vi "Create_Raw_data_file.vi"(4 "No of averages":i32=1, 5 "End time":dbl, 6 "Start time":dbl, 7 "Setup filename":string) -> (0 "Error String":string, 1 "Values":string[][](array[string]), 2 "Header Comments":string[](array[string]), 3 "Column headers":string[](array[string]))   [LabVIEW 2011]
uses:
  File/Setup_Filetype.ctl
  Controls/Post_Process.ctl
  Globals/Preference_global.vi
  Globals/Meas_global.vi
  Globals/Trav_pos_global.vi
  Globals/Constants_global.vi
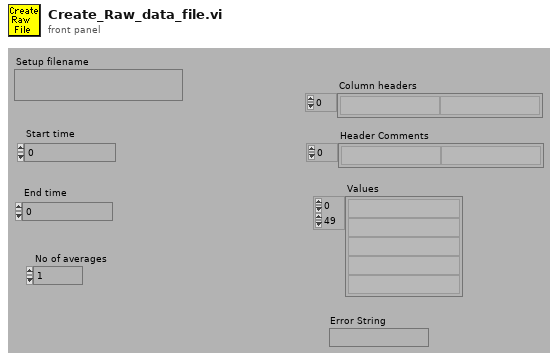
[diagram p1: front panel]
types:
  T1 = typedef "Post_Process.ctl" = enum16{"Take New Data", "Post Process Raw Data File"}
  T2 = typedef "Server_Comms.ctl" = enum16{"Server Link Healthy", "Do Not Link To Server"}
  T3 = typedef "Setup_Filetype.ctl" = enum16{"Measurement Setups", "Calibration Setups", "General", "Results File Plotter Setups", "Speed Calib Tweaks"}
  T4 = typedef "Traverse_cluster.ctl" = cluster{"Start X":dbl, "Start Y":dbl, "Start Z":dbl, "End X":dbl, "End Y":dbl, "End Z":dbl, "No. of pts.":i32, "Spacing":T5, "Filename":path, "Tunnel Speed":dbl, "Averaging time (min)":dbl, "Extra Commands":string, "Specific Arguments":string, "Emission Rate (l/min)":dbl, "Trace Gas Concentration (%)":dbl, "Density Ratio":string, "Comments":string, "Row No":i32, "Row Type Selector":T6, "Completion time":string, "Row Duration (mins)":dbl, "No. of Valid pts.":i32, "Meas Setup File":string}
  T5 = typedef "Spacing.ctl" = enum16{"Linear", "Log", "Gauss", "Specified", "N/A"}
  T6 = typedef "Multi_run_mode.ctl" = enum16{"Move Traverse Only", "Set Tunnel Speed Only", "Set Source Only", "Set Measurement Conditions", "Single Measurement", "Vertical Profile", "Lateral Profile", "Longitudinal Profile", "Explore Volume", "Multi-Axis Profile", "Auto Calibrate", "Meas Fast FID Bkgnd", "Check Beam Power", "Scanning Valve Measurement", "Run VI Named:", "Set ADAM Ch", "Wait (minutes)", "Send Message", "Synchronize With:", "Fall Back to this Row", "Turn Off Row Repeating", "Blank Row"}
  T7 = cluster{"Name":string, "X":dbl, "Y":dbl, "Z":dbl}[]
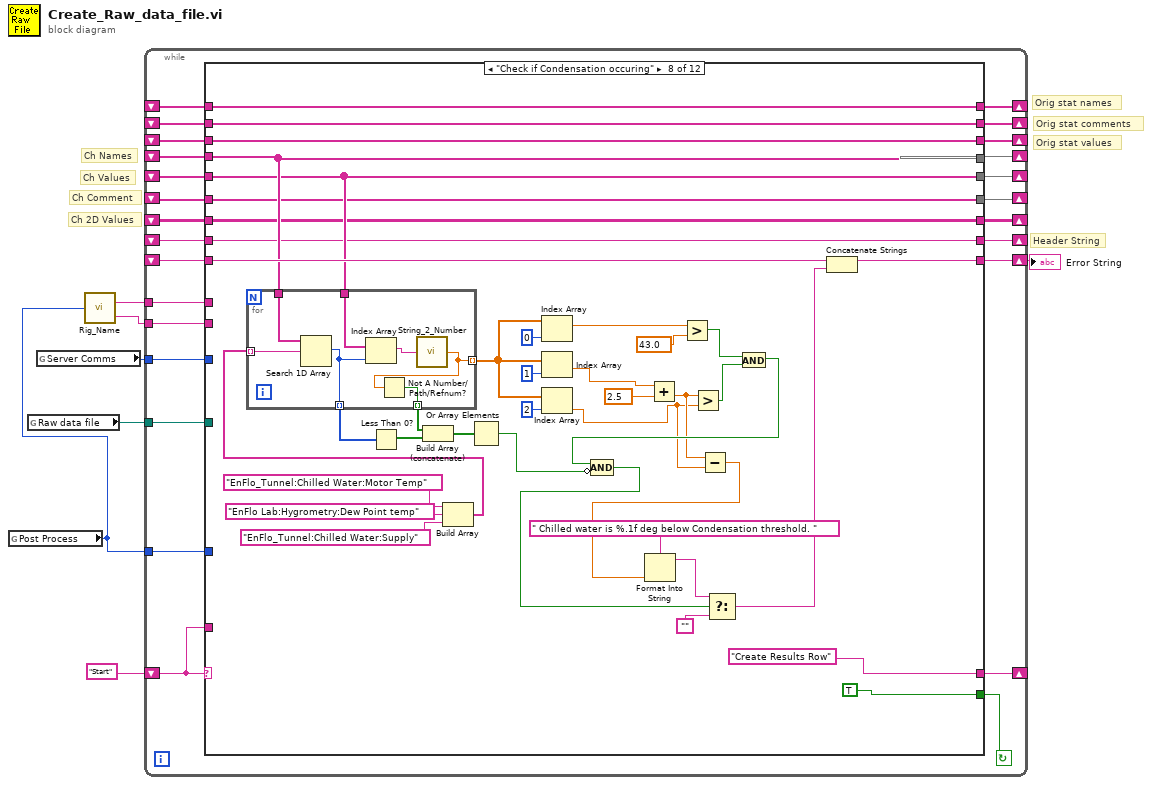
[diagram p0: block diagram]
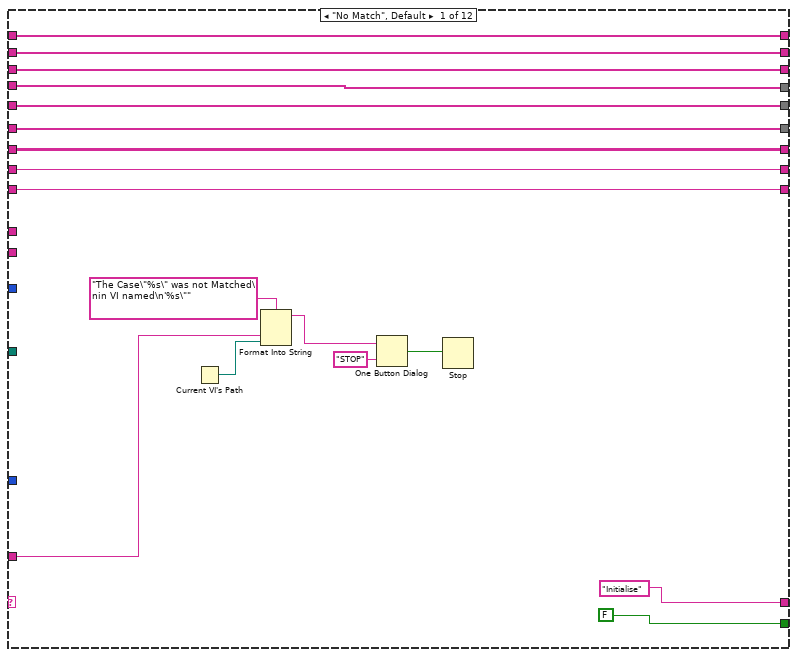
[diagram p2: hidden frame]
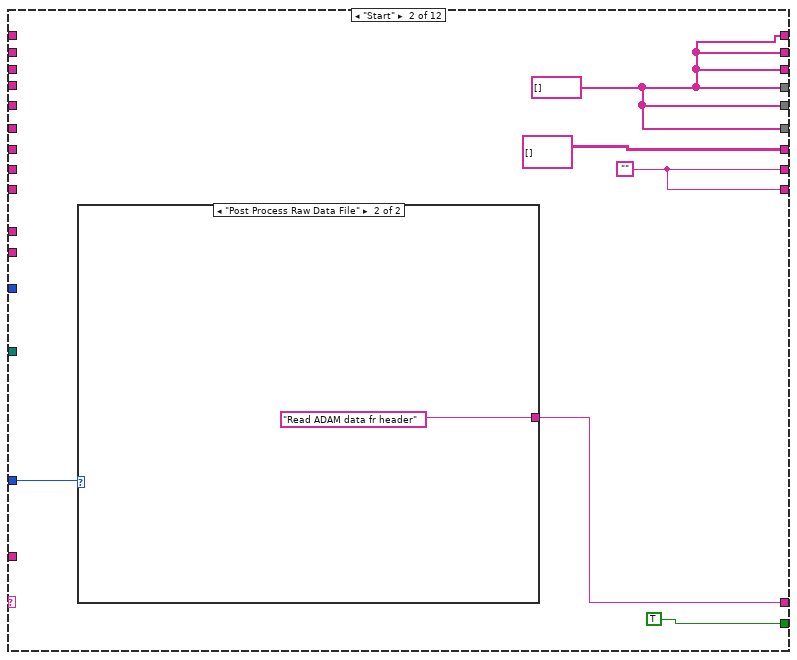
[diagram p3: hidden frame]
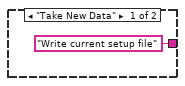
[diagram p4: hidden frame]
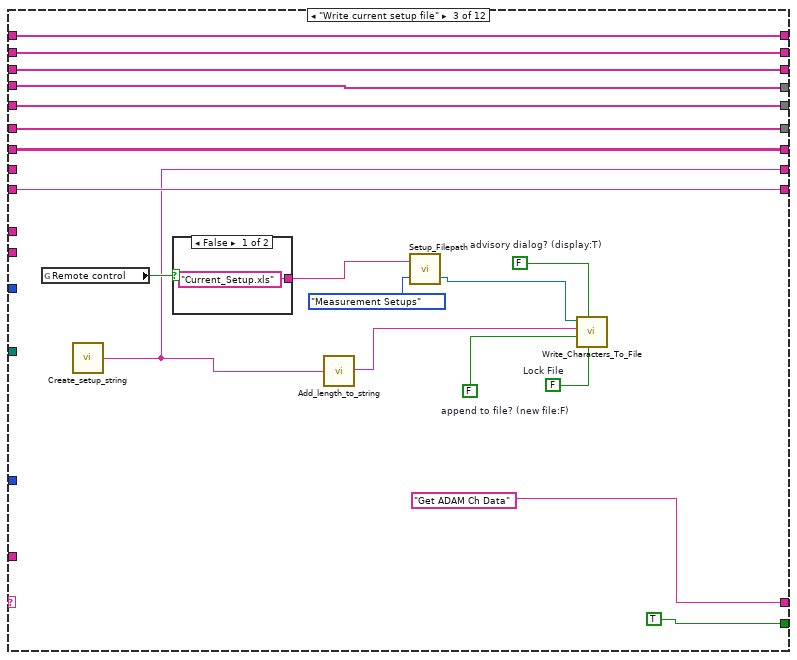
[diagram p5: hidden frame]
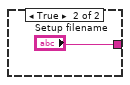
[diagram p6: hidden frame]
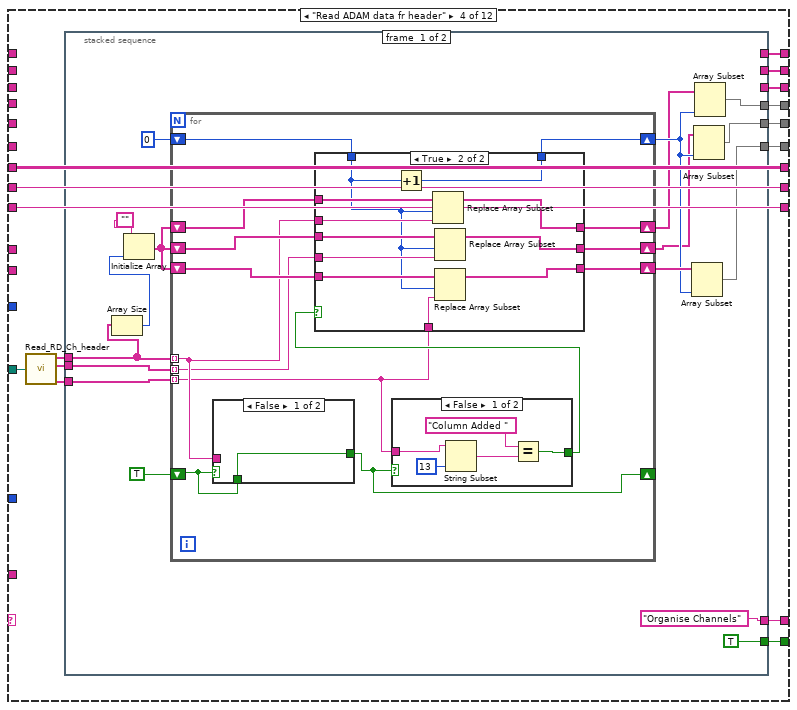
[diagram p7: hidden frame]
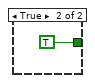
[diagram p9: hidden frame]
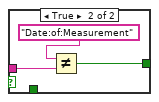
[diagram p10: hidden frame]
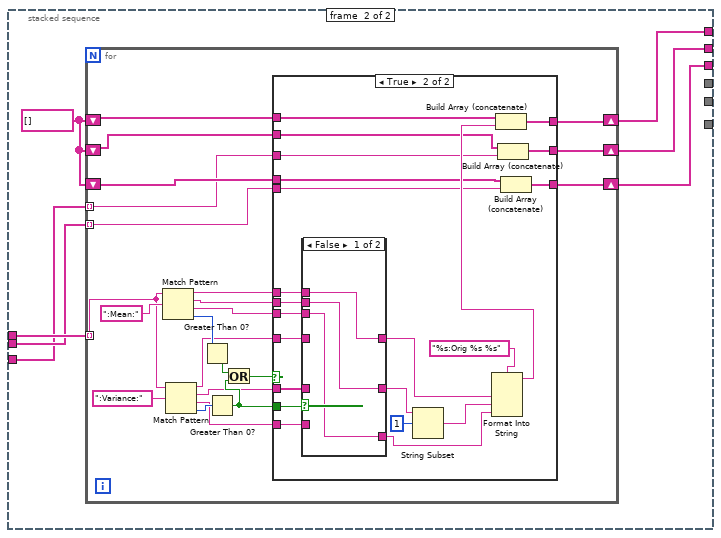
[diagram p11: hidden frame]
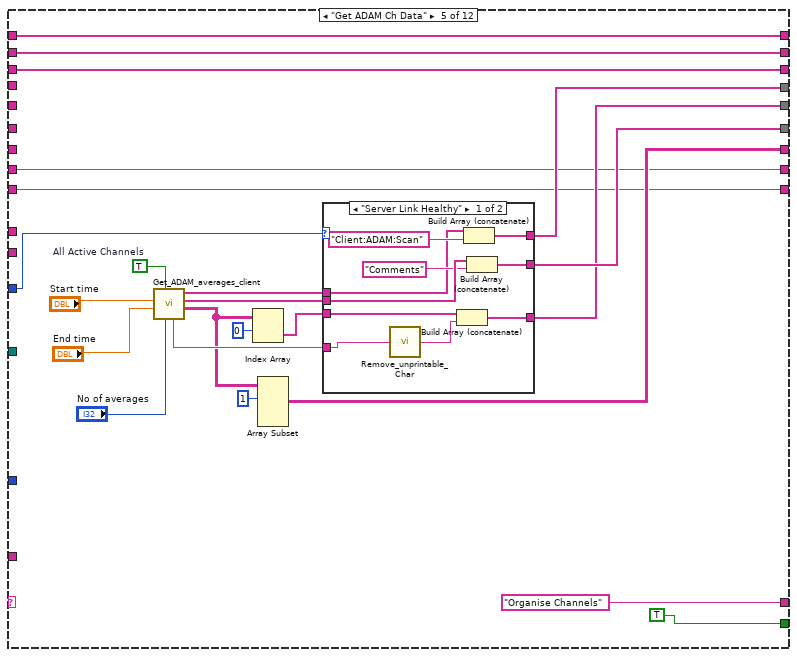
[diagram p14: hidden frame]
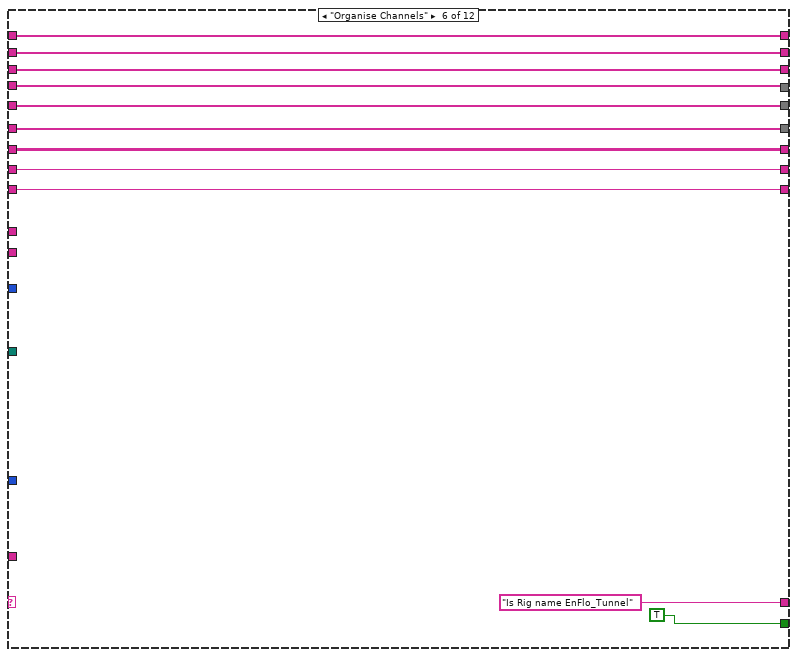
[diagram p16: hidden frame]
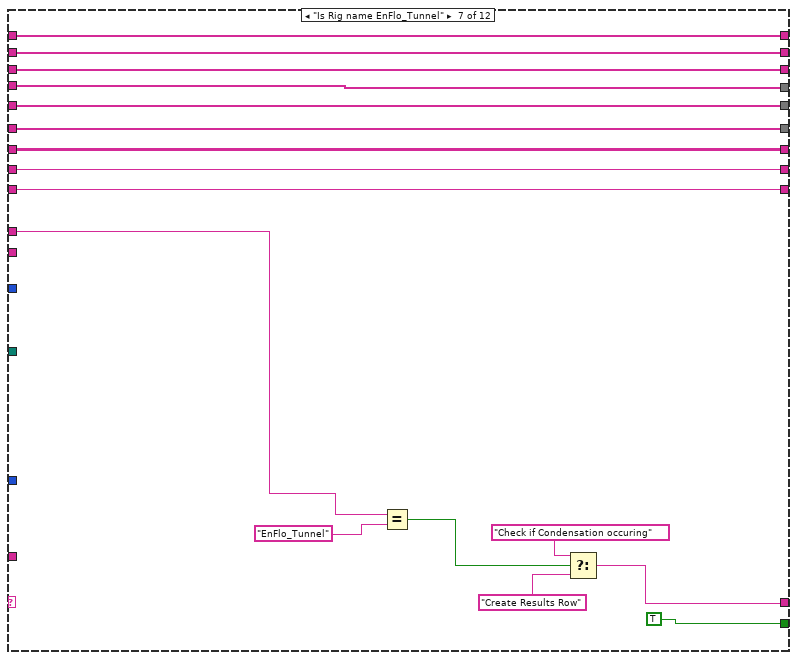
[diagram p17: hidden frame]
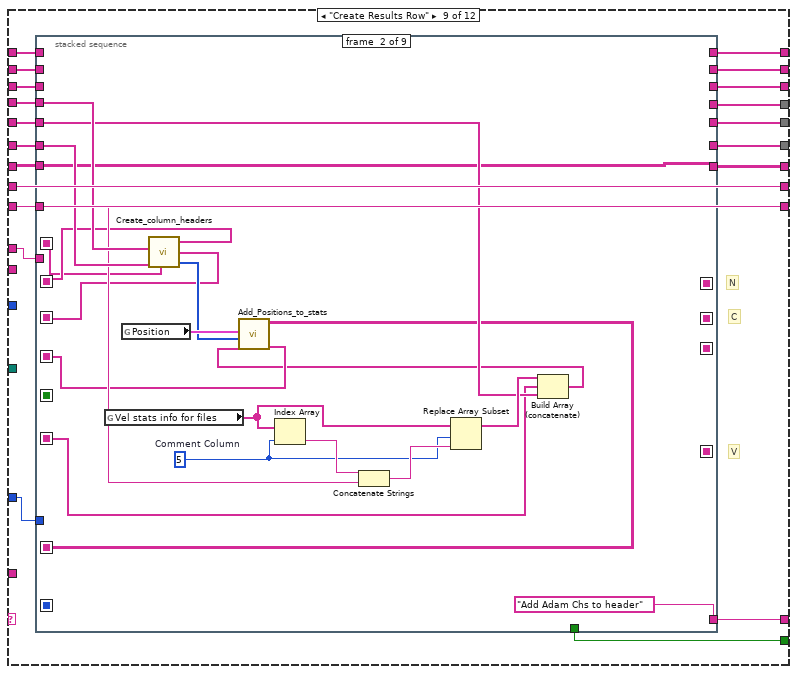
[diagram p18: hidden frame]
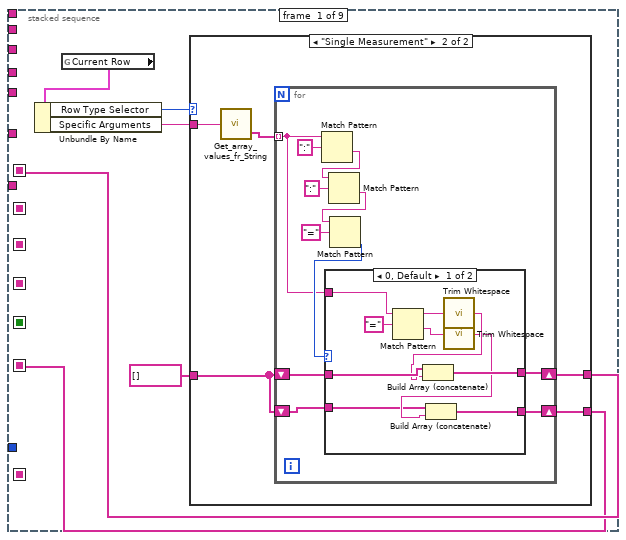
[diagram p19: hidden frame]
diagram:
  # "Orig stat values"
  # "Orig stat comments"
  # "Orig stat names"
  # "Header String"
  # "Ch 2D Values"
  # "Ch Comment"
  # "Ch Values"
  # "Ch Names"
  n1 = global read "Meas_global.vi" "Post Process"() -> (w3:T1)
  n2 = global read "Meas_global.vi" "Raw data file"() -> (w6:path)
  n3 = global read "Preference_global.vi" "Server Comms"() -> (w5:T2)
  n4 = call "Rig_Name.vi"("Post Process"=w3) -> ("Rig Setup before dash"=w2:string, "Hard Disk name"=w1:string)
  n5 = while {
    tunnel: w5 -> [w16]
    tunnel: w6 -> [w17]
    tunnel: w3 -> [w18]
    shift-left: _ -> [w20]
    shift-right: [w19] -> _
    shift-left: _ -> [w26]
    shift-right: [w25] -> w4
    shift-left: _ -> [w21]
    shift-right: [w27] -> _
    shift-left: _ -> [w22]
    shift-right: [w29] -> _
    shift-left: _ -> [w23]
    shift-right: [w28] -> _
    shift-left: _ -> [w24]
    shift-right: [w30] -> _
    shift-left: "Start" -> [w31]
    shift-right: [w32] -> _
    tunnel: w2 -> [w15]
    tunnel: w1 -> [w14]
    shift-right: [w10] -> _
    shift-left: _ -> [w11]
    shift-right: [w8] -> _
    shift-left: _ -> [w9]
    shift-right: [w12] -> _
    shift-left: _ -> [w13]
    stop <- w33 continue-if-true
    n6 = case shown="\"Check if Condensation occuring\"" w31 {
      tunnel: [FALSE TRUE TRUE w83 TRUE TRUE TRUE TRUE w328 TRUE TRUE FALSE] -> w33
      tunnel: ["Initialise" w52 "Get ADAM Ch Data" w94 "Organise Channels" "Is Rig name EnFlo_Tunnel" w265 "Create Results Row" w340 "Add Raw Data header info" "Add Raw Data fr Tempory file" "End"] -> w32
      tunnel: w31 -> [w45 _ _ _ _ _ _ _ _ _ _ _]
      tunnel: [w42 w51 w77 w85 w221 w255 w273 w283 w337 w610 w640 w657] -> w30
      tunnel: [w40 w51 w75 w86 w220 w253 w271 w281 w334 w621 w642 w659] -> w29
      tunnel: [w41 w51 w76 w84 w219 w254 w272 w282 w330 w622 w641 w658] -> w28
      tunnel: [w39 string[][] [] w74 w92 w217 w252 w270 w280 w332 w613 w643 w660] -> w27
      tunnel: w26 -> [w38 _ w72 w93 w216 w250 w267 w286 w338 w626 w644 w661]
      tunnel: [w38 w54 w72 w93 w216 w250 w267 w284 w338 w626 w644 w661] -> w25
      tunnel: w24 -> [w42 _ w77 _ _ w255 w273 w283 w336 w610 w640 w657]
      tunnel: w23 -> [w41 _ w76 _ _ w254 w272 w282 w331 w622 w641 w658]
      tunnel: w22 -> [w40 _ w75 _ _ w253 w271 w281 w335 w621 w642 w659]
      tunnel: w21 -> [w39 _ w74 w92 _ w252 w270 w280 w333 w613 w643 w660]
      tunnel: w20 -> [w37 _ _ w91 w215 w251 w268 w278 w339 w615 w637 w656]
      tunnel: [w37 w54 w66 w91 w215 w251 w268 w278 w339 w618 w636 ""] -> w19
      tunnel: w18 -> [_ w53 _ _ _ _ _ _ w329 _ _ _]
      tunnel: w17 -> [_ _ _ w90 _ _ _ _ _ _ _ w652]
      tunnel: w16 -> [_ _ _ _ w214 _ _ _ _ _ _ _]
      tunnel: w15 -> [_ _ _ _ _ _ w262 _ w327 _ _ _]
      tunnel: w14 -> [_ _ _ _ _ _ _ _ _ _ _ _]
      tunnel: w13 -> [w36 _ w64 _ w213 w249 w260 w277 w325 w607 w635 w649]
      tunnel: [w36 w51 w64 w82 w213 w249 w260 w277 w326 w607 w635 w649] -> w12
      tunnel: w11 -> [w35 _ w63 _ w212 w248 w259 w276 w324 w606 w634 w648]
      tunnel: [w35 w51 w63 w81 w212 w248 w259 w276 w323 w606 w634 w648] -> w10
      tunnel: w9 -> [w34 _ w62 _ w211 w247 w258 w275 w321 w605 w633 w647]
      tunnel: [w34 w51 w62 w80 w211 w247 w258 w275 w322 w605 w633 w647] -> w8
      frame "No Match", Default {
        n7 = Current VI's Path() -> (path=w44:path)
        n8 = Format Into String(format string="The Case\"%s\" was not Matched\nin VI named\n'%s\"" ("Format String"), w45, w44) -> (resulting string=w48:string)  [unwired: 2 in, 1 out]
        n9 = One Button Dialog(message=w48, button name ("OK")="STOP") -> (true=w46:bool)
        n10 = Stop(stop? (T)=w46) -> ()
      }
      frame "Start" {
        w54 = ""
        w51 = string[] []
        n11 = case shown="\"Post Process Raw Data File\"" w53 {
          tunnel: ["Write current setup file" "Read ADAM data fr header"] -> w52
          frame "Take New Data" {
          }
          frame "Post Process Raw Data File" {
          }
        }
      }
      frame "Write current setup file" {
        w67 = FALSE  # Lock File
        w70 = FALSE  # advisory dialog? (display:T)
        w71 = FALSE  # append to file? (new file:F)
        n12 = global read "Meas_global.vi" "Remote control"() -> (w69:bool)
        n13 = call "Create_setup_string.vi"() -> ("Setup String"=w66:string)  [unwired: 1 out]
        n14 = case shown="False" w69 {
          tunnel: ["Current_Setup.xls" ("Setup filename") "Setup filename"] -> w60
          frame False {
          }
          frame True {
          }
        }
        n15 = call "Add_length_to_string.vi"("String in"=w66) -> ("String out"=w68:string)
        n16 = call "Setup_Filepath.vi"("Setup File Type"=Setup_Filetype."Measurement Setups", "Filename in"=w60) -> ("Filename Out"=w59:path)  [unwired: 1 out]
        n17 = call "Write_Characters_To_File.vi"("file path (dialog if empty)"=w59, "advisory dialog? (display:T)"=w70, "character string"=w68, "append to file? (new file:F)"=w71, "Lock File"=w67) -> ()  [unwired: 4 out]
      }
      frame "Read ADAM data fr header" {
        n18 = call "Read_RD_Ch_header.vi"("Raw data file"=w90) -> ("Ch Name Out"=w88:string[], "Ch Values"=w87:string[], "Comments"=w89:string[])  [unwired: 1 out]
        n19 = stacked-sequence {
          tunnel: ["Organise Channels" _] -> w94
          tunnel: w89 -> [w109 w154]
          tunnel: w88 -> [w108 w157]
          tunnel: w87 -> [w103 w155]
          tunnel: [w100 _] -> w86
          tunnel: [w97 _] -> w85
          tunnel: [w96 _] -> w84
          tunnel: [TRUE _] -> w83
          tunnel: [_ w153] -> w82
          tunnel: [_ w152] -> w81
          tunnel: [_ w151] -> w80
          frame #0 {
            n20 = Array Size(array=w108) -> (size(s)=w106:i32)
            n21 = Initialize Array("", w106) -> (w105:string[])
            n22 = for {
              shift-right: [w112] -> w101
              shift-left: 0 -> [w122]
              shift-right: [w116] -> w102
              shift-left: w105 -> [w119]
              shift-right: [w117] -> w99
              shift-left: w105 -> [w120]
              shift-right: [w118] -> w98
              shift-left: w105 -> [w121]
              shift-right: [w124] -> _
              shift-left: TRUE -> [w125]
              tunnel: w108 -> [w115] mode=indexing
              tunnel: w109 -> [w113] mode=indexing
              tunnel: w103 -> [w114] mode=indexing
              n23 = case shown="False" w125 {
                tunnel: w115 -> [_ w150]
                tunnel: [w147 w148] -> w124
                tunnel: w125 -> [w147 _]
                frame False {
                }
                frame True {
                  n24 = Not Equal?(x="Date:of:Measurement", y=w150) -> (x != y?=w148:bool)
                }
              }
              n25 = case shown="False" w124 {
                tunnel: w113 -> [w142 _]
                tunnel: [w144 TRUE] -> w123
                frame False {
                  n26 = String Subset(string=w142, length (rest)=13 ("length (rest)")) -> (substring=w141:string)  [unwired: 1 out]
                  n27 = Equal?(x="Column Added ", y=w141) -> (x = y?=w144:bool)
                }
                frame True {
                }
              }
              n28 = case shown="True" w123 {
                tunnel: w122 -> [w126 w131]
                tunnel: w121 -> [w129 w140]
                tunnel: w120 -> [w128 w139]
                tunnel: w119 -> [w127 w138]
                tunnel: [w129 w137] -> w118
                tunnel: [w128 w136] -> w117
                tunnel: [w127 w135] -> w116
                tunnel: w115 -> [_ w134]
                tunnel: w114 -> [_ w133]
                tunnel: w113 -> [_ w132]
                tunnel: [w126 w130] -> w112
                frame False {
                }
                frame True {
                  n29 = Increment(x=w131) -> (x+1=w130:i32)
                  n30 = Replace Array Subset(array=w140, new element=w134, index=w131) -> (w137:string[])
                  n31 = Replace Array Subset(array=w139, new element=w133, index=w131) -> (w136:string[])
                  n32 = Replace Array Subset(array=w138, new element=w132, index=w131) -> (w135:string[])
                }
              }
            }
            n33 = Array Subset(array=w102, length=w101) -> (w100:string[])  [unwired: 1 in]
            n34 = Array Subset(array=w99, length=w101) -> (w96:string[])  [unwired: 1 in]
            n35 = Array Subset(array=w98, length=w101) -> (w97:string[])  [unwired: 1 in]
          }
          frame #1 {
            w156 = string[] []
            n36 = for {
              shift-right: [w165] -> w153
              shift-left: w156 -> [w164]
              shift-right: [w158] -> w152
              shift-left: w156 -> [w159]
              shift-right: [w161] -> w151
              shift-left: w156 -> [w162]
              tunnel: w157 -> [w177] mode=indexing
              tunnel: w155 -> [w163] mode=indexing
              tunnel: w154 -> [w160] mode=indexing
              n37 = Match Pattern(string=w177, regular expression=":Mean:") -> (before substring=w168:string, match substring=w167:string, after substring=w166:string, offset past match=w176:i32)  [unwired: 1 out]
              n38 = Match Pattern(string=w177, regular expression=":Variance:") -> (before substring=w171:string, match substring=w170:string, after substring=w169:string, offset past match=w175:i32)  [unwired: 1 out]
              n39 = Greater Than 0?(x=w176) -> (x > 0?=w174:bool)
              n40 = Greater Than 0?(x=w175) -> (x > 0?=w172:bool)
              n41 = Or(x=w174, y=w172) -> (x .or. y?=w173:bool)
              n42 = case shown="True" w173 {
                tunnel: w172 -> [_ w204]
                tunnel: w171 -> [_ w203]
                tunnel: w170 -> [_ w202]
                tunnel: w169 -> [_ w201]
                tunnel: w168 -> [_ w194]
                tunnel: w167 -> [_ w193]
                tunnel: w166 -> [_ w192]
                tunnel: [w182 w190] -> w165
                tunnel: w164 -> [w182 w189]
                tunnel: w163 -> [_ w188]
                tunnel: w162 -> [w180 w187]
                tunnel: [w180 w186] -> w161
                tunnel: w160 -> [_ w185]
                tunnel: w159 -> [w181 w184]
                tunnel: [w181 w183] -> w158
                frame False {
                }
                frame True {
                  n43 = case shown="False" w204 {
                    tunnel: w203 -> [_ w209]
                    tunnel: w202 -> [_ w210]
                    tunnel: w201 -> [_ w208]
                    tunnel: [w206 w210] -> w199
                    tunnel: [w207 w209] -> w196
                    tunnel: [w205 w208] -> w195
                    tunnel: w194 -> [w207 _]
                    tunnel: w193 -> [w206 _]
                    tunnel: w192 -> [w205 _]
                    frame False {
                    }
                    frame True {
                    }
                  }
                  n44 = String Subset(string=w199, offset (0)=1) -> (substring=w198:string)  [unwired: 1 out]
                  n45 = Format Into String(format string="%s:Orig %s %s", w196, w198, w195) -> (resulting string=w191:string)  [unwired: 2 in, 1 out]
                  n46 = Build Array (concatenate)(w189, w191) -> (w190:string[])
                  n47 = Build Array (concatenate)(w184, w185) -> (w183:string[])
                  n48 = Build Array (concatenate)(w187, w188) -> (w186:string[])
                }
              }
            }
          }
        }
      }
      frame "Get ADAM Ch Data" {
        w224 = TRUE  # All Active Channels
        n49 = call "Get_ADAM_averages_client.vi"("No of averages"="No of averages", "All Active Channels"=w224, "End time"="End time", "Start time"="Start time") -> ("Values"=w227:string[][], "Comments"=w230:string[], "Titles"=w229:string[], "Messages"=w231:string)  [unwired: 1 in, 3 out]
        n50 = Index Array(array=w227, index (row)=0 ("Index")) -> (element=w218:string[])  [unwired: 1 in]
        n51 = Array Subset(array=w227, index (row)=1 ("Array Index")) -> (w217:string[][])  [unwired: 3 in]
        n52 = case shown="\"Server Link Healthy\"" w214 {
          tunnel: w231 -> [w235 _]
          tunnel: w230 -> [w243 w245]
          tunnel: w229 -> [w240 w246]
          tunnel: [w239 w246] -> w221
          tunnel: [w238 w245] -> w220
          tunnel: [w237 w244] -> w219
          tunnel: w218 -> [w236 w244]
          frame "Server Link Healthy" {
            n53 = call "Remove_unprintable_Char.vi"("Input String"=w235) -> ("Output String"=w234:string)
            n54 = Build Array (concatenate)(w236, w234) -> (w237:string[])
            n55 = Build Array (concatenate)(w240, "Client:ADAM:Scan") -> (w239:string[])
            n56 = Build Array (concatenate)(w243, "Comments" ("Comments")) -> (w238:string[])
          }
          frame "Do Not Link To Server" {
          }
        }
      }
      frame "Organise Channels" {
      }
      frame "Is Rig name EnFlo_Tunnel" {
        n57 = Equal?(x=w262, y="EnFlo_Tunnel") -> (x = y?=w266:bool)
        n58 = Select(t="Check if Condensation occuring", s=w266, f="Create Results Row") -> (s? t:f=w265:string)
      }
      frame "Check if Condensation occuring" {
        n59 = Build Array("EnFlo_Tunnel:Chilled Water:Motor Temp", "EnFlo Lab:Hygrometry:Dew Point temp", "EnFlo_Tunnel:Chilled Water:Supply") -> (w309:string[])
        n60 = for {
          tunnel: w283 -> [w320]
          tunnel: w309 -> [w319] mode=indexing
          tunnel: w282 -> [w318]
          tunnel: [w316] -> w310 mode=indexing
          tunnel: [w315] -> w308 mode=indexing
          tunnel: [w314] -> w301 mode=indexing
          n61 = Search 1D Array(1D array=w320, element=w319) -> (index of element=w316:i32)  [unwired: 1 out]
          n62 = Index Array(array=w318, index=w316) -> (element=w317:string)
          n63 = call "String_2_Number.vi"("Value"=w317) -> ("Numeric"=w315:dbl)
          n64 = Not A Number/Path/Refnum?(number/path/refnum=w315) -> (NaN/Path/Refnum?=w314:bool)
        }
        n65 = Less Than 0?(x=w310) -> (x < 0?=w300:bool[])
        n66 = Build Array (concatenate)(w301, w300) -> (w299:bool[])
        n67 = Or Array Elements(Boolean array=w299) -> (logical OR=w295:bool)
        n68 = Index Array(array=w308, index=0 ("Index")) -> (element=w302:dbl)
        n69 = Index Array(array=w308, index=1 ("Index")) -> (element=w298:dbl)
        n70 = Index Array(array=w308, index=2 ("Index")) -> (element=w290:dbl)
        n71 = Add(x=w298, y=2.5) -> (x+y=w291:dbl)
        n72 = Greater?(x=w302, y=43.0) -> (0:w296:bool)
        n73 = Greater?(x=w291, y=w290) -> (0:w297:bool)
        n74 = Subtract(x=w291, y=w290) -> (x-y=w289:dbl)
        n75 = Format Into String(format string=" Chilled water is %.1f deg below Condensation threshold. " ("Format String"), w289) -> (resulting string=w287:string)  [unwired: 2 in, 1 out]
        n76 = And(x=w296, y=w297) -> (x .and. y?=w294:bool)
        n77 = Compound Arithmetic op=AND(w294, invert w295) -> (w293:bool)
        n78 = Select(t=w287, s=w293, f="") -> (s? t:f=w285:string)
        n79 = Concatenate Strings(w286, w285) -> (w284:string)
      }
      frame "Create Results Row" {
        # "V"
        # "C"
        # "N"
        n80 = stacked-sequence {
          seq-local: [_ w383 _ _ _ _ _ _ _] -> [_ _ w405 w446 _ _ _ _ _]
          seq-local: [_ w382 _ _ _ _ _ _ _] -> [_ _ w401 w445 _ _ _ _ _]
          seq-local: [_ w381 _ _ _ _ _ _ _] -> [_ _ w399 w444 _ _ _ _ _]
          seq-local: [_ w378 _ _ _ _ _ _ _] -> [_ _ _ _ w481 _ _ _ _]
          seq-local: [_ _ _ w443 _ _ _ _ _] -> [_ _ _ _ w483 _ _ _ _]
          seq-local: [w342 _ _ _ _ _ _ _ _] -> [_ w377 _ _ _ _ _ _ _]
          seq-local: [w341 _ _ _ _ _ _ _ _] -> [_ w376 _ _ _ _ _ _ _]
          seq-local: [_ _ _ w442 _ _ _ _ _] -> [_ _ _ _ _ _ w538 w576 _]
          seq-local: [_ _ _ w441 _ _ _ _ _] -> [_ _ _ _ _ _ _ w574 _]
          seq-local: [_ _ _ _ w480 _ _ _ _] -> [_ _ _ _ _ _ _ w573 _]
          seq-local: [_ _ _ _ _ w498 _ _ _] -> [_ _ _ _ _ _ w537 w577 _]
          seq-local: [_ _ _ _ _ _ w536 _ _] -> [_ _ _ _ _ _ _ w575 _]
          tunnel: [_ "Add Adam Chs to header" _ _ _ _ _ _ _] -> w340
          tunnel: w336 -> [_ w394 w403 _ _ w501 _ _ _]
          tunnel: w335 -> [_ w393 w404 _ _ _ _ _ _]
          tunnel: w338 -> [_ w385 _ _ _ _ _ _ _]
          tunnel: w331 -> [_ w384 w398 _ _ w500 _ _ _]
          tunnel: w333 -> [_ w380 _ _ _ _ _ _ _]
          tunnel: [_ _ w402 _ _ _ _ _ _] -> w337
          tunnel: [_ _ w400 _ _ _ _ _ _] -> w334
          tunnel: [_ w380 _ _ _ _ _ _ _] -> w332
          tunnel: [_ _ w397 _ _ _ _ _ _] -> w330
          tunnel: w329 -> [_ _ w396 w447 _ w508 _ _ _]
          tunnel: [_ _ _ _ _ w504 _ _ _] -> w328
          tunnel: w327 -> [_ _ _ _ _ w502 _ _ _]
          tunnel: [_ _ _ _ _ _ _ _ w604] -> w326
          tunnel: w325 -> [_ _ _ _ _ _ _ w571 w604]
          tunnel: w324 -> [_ _ _ _ _ _ _ w568 w603]
          tunnel: [_ _ _ _ _ _ _ _ w603] -> w323
          tunnel: [_ _ _ _ _ _ _ _ w602] -> w322
          tunnel: w321 -> [_ _ _ _ _ _ _ w565 w602]
          frame #0 {
            n81 = global read "Trav_pos_global.vi" "Current Row"() -> (w346:T4)
            n82 = Unbundle By Name(w346) -> ("Row Type Selector"=w345:T6, "Specific Arguments"=w344:string)
            n83 = case shown="\"Single Measurement\"" w345 {
              tunnel: w344 -> [_ w352]
              tunnel: string[] [] -> [w347 w350]
              tunnel: [w347 w349] -> w342
              tunnel: [w347 w348] -> w341
              frame "Move Traverse Only", Default {
              }
              frame "Single Measurement" {
                n84 = call "Get_array_values_fr_String.vi"("String Value"=w352) -> ("String array"=w351:string[])  [unwired: 1 out]
                n85 = for {
                  tunnel: w351 -> [w355] mode=indexing
                  shift-right: [w353] -> w348
                  shift-left: w350 -> [w354]
                  shift-right: [w356] -> w349
                  shift-left: w350 -> [w357]
                  n86 = Match Pattern(string=w355, regular expression=":") -> (after substring=w361:string)  [unwired: 4 out]
                  n87 = Match Pattern(string=w361, regular expression=":") -> (after substring=w359:string)  [unwired: 4 out]
                  n88 = Match Pattern(string=w359, regular expression="=") -> (offset past match=w358:i32)  [unwired: 4 out]
                  n89 = case shown="0, Default" w358 {
                    tunnel: w357 -> [w373 w375]
                    tunnel: [w372 w375] -> w356
                    tunnel: w355 -> [w368 _]
                    tunnel: w354 -> [w365 w374]
                    tunnel: [w364 w374] -> w353
                    frame 0, Default {
                      n90 = Match Pattern(string=w368, regular expression="=") -> (before substring=w370:string, after substring=w369:string)  [unwired: 3 out]
                      n91 = call <vilib>:"Trim Whitespace.vi"("string"=w370) -> ("trimmed string"=w367:string)  [unwired: 1 in]
                      n92 = Build Array (concatenate)(w373, w367) -> (w372:string[])
                      n93 = call <vilib>:"Trim Whitespace.vi"("string"=w369) -> ("trimmed string"=w366:string)  [unwired: 1 in]
                      n94 = Build Array (concatenate)(w365, w366) -> (w364:string[])
                    }
                    frame -1 {
                    }
                  }
                }
              }
            }
          }
          frame #1 {
            w386 = 5  # Comment Column
            n95 = global read "Meas_global.vi" "Vel stats info for files"() -> (w387:string[])
            n96 = global read "Meas_global.vi" "Position"() -> (w392:T7)
            n97 = call "Create_column_headers.vi"("ADAM Titles"=w394, "ADAM Comments"=w393, "Additional Channels"=w377) -> ("Column headers"=w383:string[], "Header Comments"=w382:string[], "No of stats columns"=w391:i32[])  [unwired: 2 out]
            n98 = Index Array(array=w387, index=w386) -> (element=w389:string)
            n99 = Concatenate Strings(w389, w385) -> (w390:string)
            n100 = Replace Array Subset(array=w387, new element=w390, index=w386) -> (w388:string[])
            n101 = Build Array (concatenate)(w388, w376, w384) -> (w379:string[])
            n102 = call "Add_Positions_to_stats.vi"("Data row"=w379, "No of stats columns"=w391, "Position"=w392) -> ("Data row with positions"=w381:string[], "row splitting"=w378:string[][])  [unwired: 1 in, 6 out]
          }
          frame #2 {
            n103 = case shown="\"Take New Data\"" w396 {
              tunnel: w405 -> [w414 _]
              tunnel: w404 -> [w413 w439]
              tunnel: w403 -> [w412 w440]
              tunnel: [w411 w440] -> w402
              tunnel: w401 -> [w410 _]
              tunnel: [w409 w439] -> w400
              tunnel: w399 -> [w408 _]
              tunnel: w398 -> [w407 w438]
              tunnel: [w406 w438] -> w397
              frame "Take New Data" {
                n104 = for {
                  tunnel: w412 -> [w425]
                  tunnel: w414 -> [w421] mode=indexing
                  shift-right: [w422] -> w411
                  shift-left: w412 -> [w423]
                  shift-right: [w419] -> w409
                  shift-left: w413 -> [w420]
                  shift-right: [w416] -> w406
                  shift-left: w407 -> [w417]
                  tunnel: w410 -> [w418] mode=indexing
                  tunnel: w408 -> [w415] mode=indexing
                  n105 = Search 1D Array(1D array=w425, element=w421) -> (index of element=w424:i32)  [unwired: 1 out]
                  n106 = case shown="-1" w424 {
                    tunnel: w423 -> [w428 w437]
                    tunnel: [w428 w435] -> w422
                    tunnel: w421 -> [_ w436]
                    tunnel: w420 -> [w427 w434]
                    tunnel: [w427 w433] -> w419
                    tunnel: w418 -> [_ w432]
                    tunnel: w417 -> [w426 w430]
                    tunnel: [w426 w429] -> w416
                    tunnel: w415 -> [_ w431]
                    frame 0, Default {
                    }
                    frame -1 {
                      n107 = Build Array (concatenate)(w430, w431) -> (w429:string[])
                      n108 = Build Array (concatenate)(w437, w436) -> (w435:string[])
                      n109 = Build Array (concatenate)(w434, w432) -> (w433:string[])
                    }
                  }
                }
              }
              frame "Post Process Raw Data File" {
              }
            }
          }
          frame #3 {
            # "Values"
            # "Comments"
            # "Ch Names"
            n110 = case shown="\"Post Process Raw Data File\"" w447 {
              tunnel: [w450 w456] -> w442
              tunnel: w446 -> [w450 w457]
              tunnel: [w449 w455] -> w441
              tunnel: w445 -> [w449 w453]
              tunnel: [w448 w454] -> w443
              tunnel: w444 -> [w448 w452]
              frame "Take New Data" {
              }
              frame "Post Process Raw Data File" {
                w451 = string[] []
                n111 = for {
                  shift-right: [w465] -> w456
                  shift-left: w451 -> [w466]
                  shift-right: [w460] -> w455
                  shift-left: w451 -> [w463]
                  shift-right: [w461] -> w454
                  shift-left: w451 -> [w462]
                  tunnel: w457 -> [w464] mode=indexing
                  tunnel: w453 -> [w459] mode=indexing
                  tunnel: w452 -> [w458] mode=indexing
                  n112 = Search 1D Array(1D array=w466, element=w464) -> (index of element=w467:i32)  [unwired: 1 out]
                  n113 = case shown="-1" w467 {
                    tunnel: w466 -> [w470 w479]
                    tunnel: [w470 w478] -> w465
                    tunnel: w464 -> [_ w477]
                    tunnel: w463 -> [w469 w476]
                    tunnel: w462 -> [w468 w475]
                    tunnel: [w468 w474] -> w461
                    tunnel: [w469 w473] -> w460
                    tunnel: w459 -> [_ w472]
                    tunnel: w458 -> [_ w471]
                    frame 0, Default {
                    }
                    frame -1 {
                      n114 = Build Array (concatenate)(w479, w477) -> (w478:string[])
                      n115 = Build Array (concatenate)(w476, w472) -> (w473:string[])
                      n116 = Build Array (concatenate)(w475, w471) -> (w474:string[])
                    }
                  }
                }
              }
            }
          }
          frame #4 {
            n117 = Array Size(array=w481) -> (size(s)=w486:i32[])
            n118 = Index Array(array=w486, index=0) -> (element=w484:i32)
            n119 = Greater Than 0?(x=w484) -> (x > 0?=w482:bool)
            n120 = case shown="True" w482 {
              tunnel: w483 -> [w488 w492]
              tunnel: w481 -> [_ w490]
              tunnel: [w487 w489] -> w480
              frame False {
                n121 = Build Array(w488) -> (w487:string[][])
              }
              frame True {
                n122 = Search 1D Array(1D array=w492, element="Instrument_name_place_holder") -> (index of element=w491:i32)  [unwired: 1 out]
                n123 = for {
                  tunnel: w492 -> [w497]
                  tunnel: w491 -> [w496]
                  tunnel: w490 -> [w495] mode=indexing
                  tunnel: [w494] -> w489 mode=indexing
                  n124 = Replace Array Subset(array=w497, new element=w495, index=w496) -> (w494:string[])
                }
              }
            }
          }
          frame #5 {
            n125 = Equal?(x="EnFlo_Tunnel", y=w502) -> (x = y?=w499:bool)
            n126 = case shown="True" w499 {
              tunnel: w501 -> [_ w517]
              tunnel: w500 -> [_ w514]
              tunnel: [FALSE w512] -> w498
              frame False {
              }
              frame True {
                n127 = disable-structure shown="Enabled" {
                  disable-tunnel: [w518 FALSE] -> w510
                  frame Disabled {
                    n128 = global read "Meas_global.vi" "Pre Setup String"() -> (w522:string)
                    n129 = call "Get_Characters_from_string.vi"("Input string"=w522, "Variable name"="Show_all_EnFlo_Tunnel_Columns") -> ("Status"=w520:enum16{"Char in string", "Char not in string"}, "Value"=w519:string)  [unwired: 1 in]
                    n130 = case shown="\"Char in string\"" w520 {
                      tunnel: w519 -> [w525 _]
                      tunnel: [w523 TRUE] -> w518
                      frame "Char in string" {
                        n131 = Equal?(x=w525, y="TRUE") -> (x = y?=w524:bool)
                        n132 = Not(x=w524) -> (.not. x?=w523:bool)
                      }
                      frame "Char not in string" {
                      }
                    }
                  }
                  frame Enabled {
                  }
                }
                n133 = Search 1D Array(1D array=w517, element="EnFlo_Tunnel:Heater:Enable") -> (index of element=w515:i32)  [unwired: 1 out]
                n134 = case shown="-1" w515 {
                  tunnel: w515 -> [w534 _]
                  tunnel: w514 -> [w533 _]
                  tunnel: [w529 FALSE] -> w513
                  frame 0, Default {
                    n135 = Index Array(array=w533, index=w534) -> (element=w532:string)
                    n136 = call "String_2_Number.vi"("Value"=w532) -> ("Numeric"=w531:dbl)
                    n137 = Less?(x=w531, y=0.5) -> (x < y?=w529:bool)
                  }
                  frame -1 {
                  }
                }
                n138 = Select(t=w513, s=w510, f=FALSE) -> (s? t:f=w512:bool)
              }
            }
            n139 = global read "Trav_pos_global.vi" "Dummy Measurement?"() -> (w505:bool)
            n140 = Equal?(x=Post_Process."Take New Data" ("Post Process"), y=w508) -> (x = y?=w506:bool)
            n141 = Compound Arithmetic op=AND(invert w505, w506) -> (w504:bool)
          }
          frame #6 {
            n142 = case shown="True" w537 {
              tunnel: w538 -> [_ w544]
              tunnel: [i32[] [] w542] -> w536
              frame False {
              }
              frame True {
                w540 = string[] ["EnFlo_Tunnel:Inlet Heater:Temp", "EnFlo_Tunnel:Inlet Rake:Temp", "EnFlo_Tunnel:Trav Thermo:", "EnFlo_Tunnel:floor ", "EnFlo_Tunnel:roof ", "EnFlo_Tunnel:Side ", "EnFlo_Tunnel:Temp:Inlet", "EnFlo_Tunnel:Temp:Floor"] ("Column headers")
                # "Remove these\nChannels"
                # "Remaining\nChannels"
                n143 = for {
                  tunnel: w540 -> [w546] mode=indexing
                  tunnel: [w545] -> w541 mode=indexing
                  n144 = String Length(string=w546) -> (length=w545:i32)
                }
                n145 = for {
                  tunnel: w544 -> [w550] mode=indexing
                  shift-right: [w553] -> w542
                  shift-left: i32[] [] -> [w554]
                  tunnel: w541 -> [w551]
                  tunnel: w540 -> [w549]
                  i -> [w552]
                  n146 = for {
                    tunnel: w551 -> [w559] mode=indexing
                    tunnel: w550 -> [w558]
                    tunnel: w549 -> [w556] mode=indexing
                    tunnel: [w555] -> w548 mode=indexing
                    n147 = String Subset(string=w558, length (rest)=w559) -> (substring=w557:string)  [unwired: 1 out]
                    n148 = Equal?(x=w557, y=w556) -> (x = y?=w555:bool)
                  }
                  n149 = Or Array Elements(Boolean array=w548) -> (logical OR=w547:bool)
                  n150 = case shown="True" w547 {
                    tunnel: w554 -> [w562 w563]
                    tunnel: w552 -> [w561 _]
                    tunnel: [w560 w563] -> w553
                    frame False {
                      n151 = Build Array (concatenate)(w562, w561) -> (w560:i32[])
                    }
                    frame True {
                    }
                  }
                }
              }
            }
          }
          frame #7 {
            n152 = case shown="True" w577 {
              tunnel: w576 -> [w583 w590]
              tunnel: w575 -> [_ w585]
              tunnel: w574 -> [w582 w589]
              tunnel: [w583 w588] -> w572
              tunnel: [w582 w587] -> w569
              tunnel: w573 -> [w581 w586]
              tunnel: [w581 w584] -> w566
              frame False {
              }
              frame True {
                n153 = for {
                  tunnel: w586 -> [w593] mode=indexing
                  tunnel: w585 -> [w592]
                  tunnel: [w591] -> w584 mode=indexing
                  n154 = for {
                    tunnel: w593 -> [w595]
                    tunnel: w592 -> [w596] mode=indexing
                    tunnel: [w594] -> w591 mode=indexing
                    n155 = Index Array(array=w595, index=w596) -> (element=w594:string)
                  }
                }
                n156 = for {
                  tunnel: w590 -> [w601]
                  tunnel: w585 -> [w597] mode=indexing
                  tunnel: w589 -> [w600]
                  tunnel: [w599] -> w588 mode=indexing
                  tunnel: [w598] -> w587 mode=indexing
                  n157 = Index Array(array=w600, index=w597) -> (element=w598:string)
                  n158 = Index Array(array=w601, index=w597) -> (element=w599:string)
                }
              }
            }
            n159 = for {
              tunnel: w566 -> [w580] mode=indexing
              tunnel: w565 -> [w579]
              tunnel: [w578] -> w564 mode=indexing
              n160 = Build Array (concatenate)(w580, w579) -> (w578:string[])
            }
            "Values" <- w564
            n161 = Build Array (concatenate)(w572, w571) -> (→"Column headers":string[])
            n162 = Build Array (concatenate)(w569, w568) -> (→"Header Comments":string[])
          }
          frame #8 {
          }
        }
      }
      frame "Add Adam Chs to header" {
        w608 = FALSE  # Email On Error?
        n163 = call "Channel_name_checker.vi"("Email On Error?"=w608, "Channel names"=w610) -> ("Channel names Out"=w609:string[])  [unwired: 1 out]
        n164 = for {
          tunnel: w609 -> [w632] mode=indexing
          tunnel: [w631] -> w625 mode=indexing
          tunnel: [w630] -> w624 mode=indexing
          tunnel: [w629] -> w623 mode=indexing
          n165 = call "Split_Ch_name.vi"("Ch name"=w632) -> ("Top level"=w631:string, "Middle"=w630:string, "Low level"=w629:string)
        }
        n166 = Array To Spreadsheet String(array=w613, 3:"%s" ("format string")) -> (spreadsheet string=w611:string)  [unwired: 1 out]
        n167 = Build Array(w625, w624, w623, w622, w621) -> (w619:string[][])
        n168 = Array To Spreadsheet String(array=w619, 3:"%s" ("format string")) -> (spreadsheet string=w612:string)  [unwired: 1 out]
        n169 = Concatenate Strings(w612, w611, "***************************************" ("Substring"), "\r", w615) -> (w618:string)
      }
      frame "Add Raw Data header info" {
        n170 = String Length(string=w637) -> (length=w639:i32)
        n171 = call "Raw_Data_File_Start_text.vi"("Header length"=w639) -> ("Start String"=w638:string)
        n172 = Concatenate Strings(w638, w637) -> (w636:string)
      }
      frame "Add Raw Data fr Tempory file" {
        w650 = 0  # Start to copy file at:
        n173 = global read "Constants_global.vi" "Data Folder Local"() -> (w654:path)
        n174 = Build Path(base path=w654, name or relative path="Tempory_Raw_Data_File.xls") -> (appended path=w651:path)
        n175 = call "Piece_file_Copy.vi"("File Start String"=w656, "Start to copy file at:"=w650, "Source File"=w651, "Target File"=w652) -> ()  [unwired: 1 out]
      }
    }
  }
  "Error String" <- w4
